vi "niFPGA SQRT Integer (64 bit) - Rounded.vi"(4 "x [U64]":u64 format="%.0x") -> (1 "sqrt (x) [U32]":u32 format="%.0x")   [LabVIEW 2017]
doc: "Iteratively computes the rounded integer square root of an unsigned 64-bit input using a binary restoring square root extraction algorithm. The rounding mode is round to nearest (+Inf), in which one extra bit is computed to determine whether to round up or down.\n\nNOTE: Input values must be less than (2^32 - .5)^2 (ie, less than or equal to xFFFFFFFF00000000) in order to avoid overflowing the 32-bit output integer. Overflow will result in an output of zero."
uses:
  <vilib>/Platform/TimedLoop/XDataNode/timing_clust.ctl
  <vilib>/Platform/TimedLoop/XDataNode/nitl_modes.ctl
  <vilib>/Platform/TimedLoop/XDataNode/wakeup.ctl
  <vilib>/Platform/TimedLoop/XDataNode/XDataNode.xnode
  <vilib>/Platform/TimedLoop/XDataNode/XDNodeRunTimeDep.lvlib
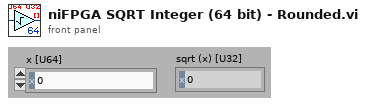
[diagram p1: front panel]
types:
  T1 = typedef "XDNodeRunTimeDep.lvlib/timing_clust.ctl" = cluster{"Expected End [f-1]":u64, "Actual End [f-1]":u64, "Finished Late? [f-1]":bool, "Expected End [i-1]":u64, "Actual End [i-1]":u64, "Finished Late? [i-1]":bool, "Expected Start [i]":u64, "Actual Start [i]":u64, "Expected Start [f]":u64, "Actual Start [f]":u64, "Source Name":string, "Structure Name":string, "Period":i64, "Deadline":i64, "Offset":i64, "Start":i64, "Priority":i32, "Timeout":i32, "Mode":T2, "Wakeup Reason":T3, "Error":errorcluster, "Source Type":string, "Secondary Source Type":string, "Global End Time":u64, "Global Start Time":u64, "Frame Duration":u64, "Iteration Duration":u64, "Assigned CPU":i32, "I/O Scan Engine Mode":u32}
  T2 = typedef "XDNodeRunTimeDep.lvlib/nitl_modes.ctl" = enum32{"No Change", "Process missed periods, maintain original phase", "Discard missed periods, maintain original phase", "Process missed periods, ignore original phase", "Discard missed periods, ignore original phase"}
  T3 = typedef "XDNodeRunTimeDep.lvlib/wakeup.ctl" = enum32{"Normal", "Aborted", "Asynchronous wakeup", "Timing source error", "Timed loop error", "Timeout"}
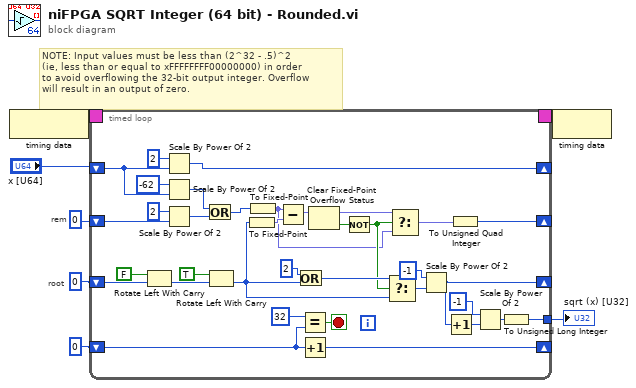
[diagram p0: block diagram]
diagram:
  # "NOTE: Input values must be less than (2^32 - .5)^2 \n(ie, less than or equal to xFFFFFFFF00000000) in order \nto avoid overflowing the 32-bit output integer. Overflow \nwill result in an output of zero."
  # "rem"
  # "root"
  n1 = node-c288() -> (w3:T1)
  n2 = timed-loop {
    timing-out: [_] -> w4
    timing: w3 -> [_]
    shift-left: u64 0 ("x [U32.2]") -> [w34]
    shift-right: [w11] -> _
    shift-left: u64 0 ("x [U32.2]") -> [w42]
    shift-right: [w14] -> _
    shift-left: "x [U64]" -> [w39]
    shift-right: [w35] -> _
    shift-right: [w19] -> _
    shift-left: u8 0 -> [w20]
    tunnel: [w13] -> w1
    stop <- w18 stop-if-true
    n3 = Rotate Left With Carry(2:w42, 3:FALSE ("carry")) -> (0:w31:u64)  [unwired: 1 out]
    n4 = Scale By Power Of 2(n=i8 2, x=w39) -> (x*2^n=w35:u64)
    n5 = Scale By Power Of 2(n=i8 -62, x=w39) -> (x*2^n=w37:u64)
    n6 = Scale By Power Of 2(n=i8 2, x=w34) -> (x*2^n=w33:u64)
    n7 = Or(x=w37, y=w33) -> (x .or. y?=w23:u64)
    n8 = Rotate Left With Carry(2:w31, 3:TRUE ("carry")) -> (0:w26:u64)  [unwired: 1 out]
    n9 = To Fixed-Point(number=w26) -> (fixed-point=w12:fxp<+,64,64>)  [unwired: 1 out]
    n10 = To Fixed-Point(number=w23) -> (fixed-point=w8:fxp<+,64,64>)  [unwired: 1 out]
    n11 = Subtract(x=w8, y=w12) -> (x-y=w24:fxp<+,64,64>)
    n12 = Or(x=u64 2, y=w26) -> (x .or. y?=w28:u64)
    n13 = Equal?(x=u8 32, y=w20) -> (x = y?=w18:bool)
    n14 = Increment(x=w20) -> (x+1=w19:u8)
    n15 = Clear Fixed-Point Overflow Status(3:w24) -> (0:w9:bool, 1:w10:fxp<+,64,64>)
    n16 = Not(x=w9) -> (.not. x?=w25:bool)
    n17 = Select(t=w28, s=w25, f=w26) -> (s? t:f=w27:u64)
    n18 = Select(t=w10, s=w25, f=w8) -> (s? t:f=w22:fxp<+,64,64>)
    n19 = Scale By Power Of 2(n=i8 -1, x=w27) -> (x*2^n=w14:u64)
    n20 = Increment(x=w14) -> (x+1=w17:u64)
    n21 = To Unsigned Quad Integer(1:w22) -> (0:w11:u64)
    n22 = Scale By Power Of 2(n=i8 -1, x=w17) -> (x*2^n=w15:u64)
    n23 = To Unsigned Long Integer(number=w15) -> (unsigned 32bit integer=w13:u32)
  }
  "sqrt (x) [U32]" <- w1
  n24 = node-c288(w4) -> ()
